vi "Add Default Buffer Converter Transfer Configuration.vi"(8 "error in":errorcluster, 10 "transfer settings":T1={"byte order"=enum."little-endian"}, 11 "transfer":T3={"core"={"name"="Transfer"}, "component settings"=[], "channels"=[]} {"channels"."core"."string offset" format="%d bytes"}) -> (0 "error out":errorcluster, 3 "transfer out":T3={"core"={"name"="Transfer"}, "component settings"=[], "channels"=[]} {"channels"."core"."string offset" format="%d bytes"})   [LabVIEW 2020, in "DSF Configuration API.lvlib"]
uses:
  DSF Configuration API.lvlib
  Includes/DSF Core.lvlibp/Typedefs/DSF Engine Transfer Configuration.ctl
  Includes/DSF Core.lvlibp/Typedefs/Core Transfer Configuration.ctl
  Includes/DSF Core.lvlibp/Typedefs/DSF Settings Info.ctl
  Includes/DSF Core.lvlibp/Typedefs/DSF Engine Channel Configuration.ctl
  Includes/DSF Core.lvlibp/Typedefs/Core Channel Configuration.ctl
  Includes/DSF Core.lvlibp/Typedefs/DSF Data Type.ctl
  Default Buffer Converter Transfer Settings.ctl
  Includes/DSF Core.lvlibp/Typedefs/DSF Byte Order.ctl
  927315ce-c5ef-419c-843f-17545a997176.vi
  Includes/DSF Core.lvlibp
  Includes/DSF Core.lvlibp/Classes/Configuration/Core/Transfer/Transfer Configuration.lvclass
  Includes/DSF Core.lvlibp/Classes/Configuration/Core/Channel/Channel Configuration.lvclass
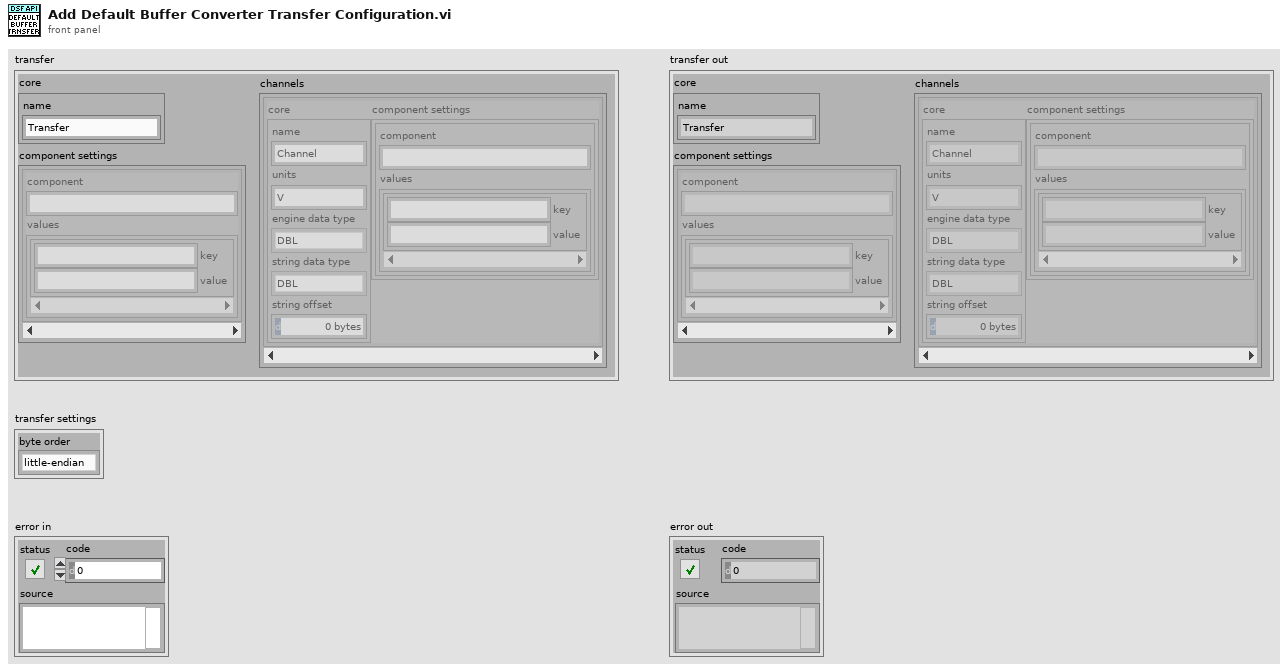
[diagram p1: front panel]
types:
  T1 = typedef "DSF Configuration API.lvlib/Default Buffer Converter Transfer Settings.ctl" = cluster{"byte order":T2}
  T2 = typedef "DSF Core.lvlibp/DSF Byte Order.ctl" = enum8{"big-endian", "little-endian"}
  T3 = typedef "DSF Core.lvlibp/DSF Engine Transfer Configuration.ctl" = cluster{"core":T4, "component settings":T5[], "channels":T6[]}
  T4 = typedef "DSF Core.lvlibp/Transfer Configuration.lvclass/Core Transfer Configuration.ctl" = cluster{"name":string}
  T5 = typedef "DSF Core.lvlibp/DSF Settings Info.ctl" = cluster{"component":string, "values":cluster{"key":string, "value":string}[]}
  T6 = typedef "DSF Core.lvlibp/DSF Engine Channel Configuration.ctl" = cluster{"core":T7, "component settings":T5[]}
  T7 = typedef "DSF Core.lvlibp/Channel Configuration.lvclass/Core Channel Configuration.ctl" = cluster{"name":string, "units":string, "engine data type":T8, "string data type":T8, "string offset":u64}
  T8 = typedef "DSF Core.lvlibp/DSF Data Type.ctl" = enum8{"Bool", "SGL", "DBL", "I8", "I16", "I32", "I64", "U8", "U16", "U32", "U64"}
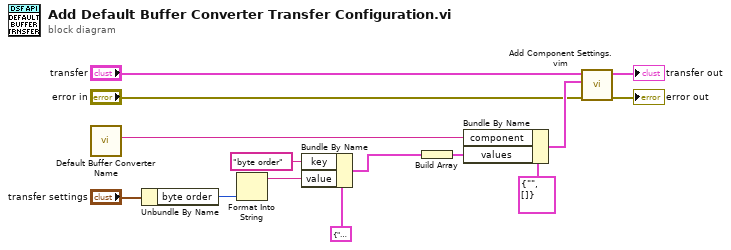
[diagram p0: block diagram]
diagram:
  n1 = call "Default Buffer Converter Name.vi"() -> ("component name"=w14:string)  [unwired: 11 in]
  n2 = Unbundle By Name("transfer settings") -> ("byte order"=w11:T2)
  n3 = Format Into String(w11) -> (resulting string=w10:string)  [unwired: 3 in, 1 out]
  n4 = Bundle By Name(cluster=cluster{"key":string, "value":string} {"key"="", "value"=""} ("setting"), "key"="byte order", "value"=w10) -> (w8:cluster{"key":string, "value":string})
  n5 = Build Array(w8) -> (w7:cluster{"key":string, "value":string}[])
  n6 = Bundle By Name(cluster=T5 {"component"="", "values"=[]} ("component settings"), "component"=w14, "values"=w7) -> (w5:T5)
  n7 = call "Add Component Settings.vim"("error in"="error in", "component settings"=w5, "dsf configuration"="transfer") -> ("error out"=→"error out":errorcluster, "dsf configuration out"=→"transfer out":T3)  [unwired: 7 in]
